vi "Compensate Digital Tach Time.vi"(7 "reset? (TRUE)":bool=TRUE, 9 "scaled signal [EU]":waveform(dbl)={"t0"=timestamp(0 s since 1904-01-01), "dt"=0.0, "Y"=[]}, 10 "initial delay[s]":dbl format="%.2f", 11 "pulse positions in[s]":dbl[](array[numeric]) format="%.2f") -> (2 "offset [s]":dbl format="%.2f", 3 "pulse positions out[s]":dbl[](array[numeric]) format="%.2f")   [LabVIEW 2017, in "SoundVib_TachProcess.lvlib"]
uses:
  <vilib>/addons/Sound and Vibration/Order Analysis/Tach Process/SoundVib_TachProcess.lvlib
  <vilib>/Waveform/WDTOps.llb/WDT Waveform Duration DBL.vi
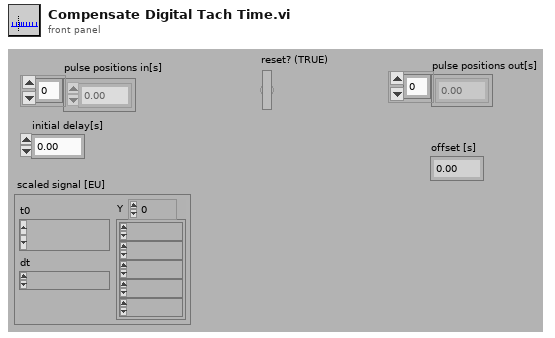
[diagram p1: front panel]
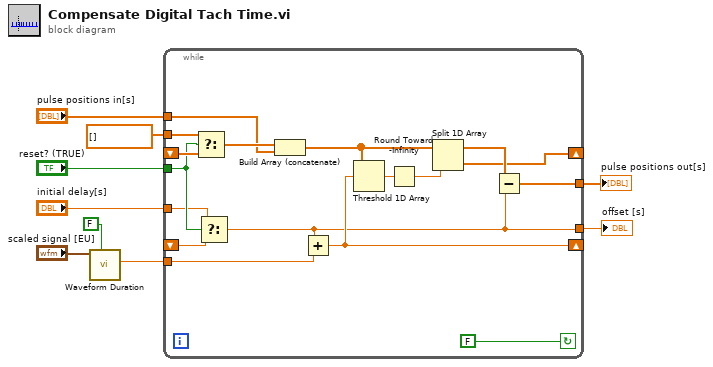
[diagram p0: block diagram]
diagram:
  n1 = call-poly <vilib>:"Waveform Duration.vi"("open interval? (T)"=FALSE, "waveform in"="scaled signal [EU]") -> ("duration"=w5:dbl)  [unwired: 7 in, 2 out]
  n2 = while {
    shift-right: [w12] -> _
    shift-left: _ -> [w24]
    shift-right: [w15] -> _
    shift-left: _ -> [w25]
    tunnel: "reset? (TRUE)" -> [w23]
    tunnel: "initial delay[s]" -> [w22]
    tunnel: w5 -> [w21]
    tunnel: "pulse positions in[s]" -> [w19]
    tunnel: [w18] -> w3
    tunnel: dbl[] [] ("t") -> [w17]
    tunnel: [w10] -> w1
    stop <- FALSE continue-if-true
    n3 = Select(t=w17, s=w23, f=w24) -> (s? t:f=w20:dbl[])
    n4 = Select(t=w22, s=w23, f=w25) -> (s? t:f=w10:dbl)
    n5 = Build Array (concatenate)(w20, w19) -> (w16:dbl[])
    n6 = Add(x=w10, y=w21) -> (x+y=w15:dbl)
    n7 = Threshold 1D Array(2:w15, 3:w16) -> (0:w14:dbl)  [unwired: 1 in]
    n8 = Round Toward -Infinity(1:w14) -> (0:w11:dbl)
    n9 = Split 1D Array(array=w16, index=w11) -> (first subarray=w13:dbl[], second subarray=w12:dbl[])
    n10 = Subtract(x=w13, y=w10) -> (x-y=w18:dbl[])
  }
  "pulse positions out[s]" <- w3
  "offset [s]" <- w1
